vi "Run.vi"(8 "error in (no error)":errorcluster, 11 "socket PUB in":refnum<class "socket PUB.lvclass">) -> (0 "error out":errorcluster, 3 "socket PUB out":refnum<class "socket PUB.lvclass">)   [LabVIEW 2018, in "socket PUB.lvclass"]
uses:
  socket PUB.lvclass
  C:/Users/Denis/Desktop/S4ACS/S4ACS/communication-manager/Socket/Socket.lvclass
  State Machine/State Machine.lvclass
  RxTx/RxTx.lvclass
  Socket/Socket.lvclass
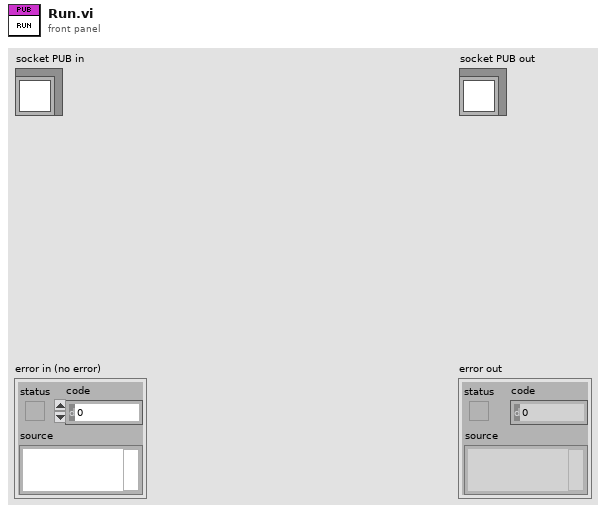
[diagram p1: front panel]
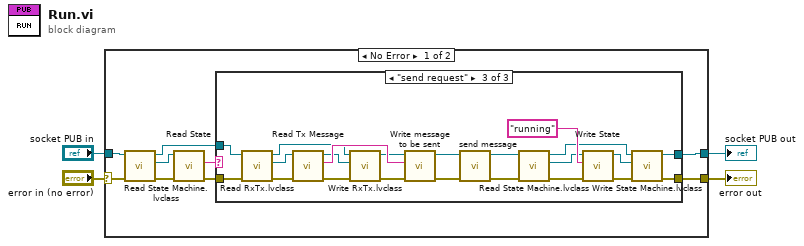
[diagram p0: block diagram]
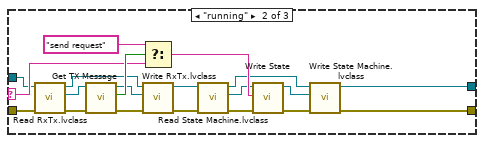
[diagram p3: hidden frame]
diagram:
  n1 = case shown="No Error" "error in (no error)" {
    selector: "error in (no error)" -> [w9 w58]
    tunnel: "socket PUB in" -> [w7 w59]
    tunnel: [w5 w59] -> w2
    tunnel: [w8 w58] -> w1
    frame No Error {
      n2 = call-dynamic "Read State Machine.lvclass.vi"("error in (no error)"=w9, "Socket in"=w7) -> ("error out"=w11:errorcluster, "State Machine.lvclass"=w13:refnum<class "State Machine.lvclass">, "Socket out"=w6:refnum<class "socket PUB.lvclass">)  [unwired: 7 in]
      n3 = call-dynamic "Read State.vi"("error in (no error)"=w11, "State Machine in"=w13) -> ("error out"=w10:errorcluster, "State"=w12:string)  [unwired: 7 in, 1 out]
      n4 = case shown="\"send request\"" w12 {
        selector: w12 -> [_ w34 _]
        tunnel: w6 -> [w15 w22 w54]
        tunnel: [w15 w16 w48] -> w5
        tunnel: [w14 w25 w47] -> w8
        tunnel: w10 -> [w14 w32 w53]
        frame Default {
        }
        frame "running" {
          n5 = call-dynamic "Read RxTx.lvclass.vi"("error in (no error)"=w32, "Socket in"=w22) -> ("error out"=w28:errorcluster, "RxTx.lvclass"=w30:refnum<class "RxTx.lvclass">, "Socket out"=w21:refnum<class "socket PUB.lvclass">)  [unwired: 7 in]
          n6 = call "Get TX Message.vi"("error in (no error)"=w28, "RxTx in"=w30) -> ("error out"=w27:errorcluster, "New msg"=w35:bool, "RxTx out"=w29:refnum<class "RxTx.lvclass">)  [unwired: 7 in]
          n7 = Select(t="send request", s=w35, f=w34) -> (s? t:f=w31:string)
          n8 = call-dynamic "Write RxTx.lvclass.vi"("error in (no error)"=w27, "RxTx.lvclass"=w29, "Socket in"=w21) -> ("error out"=w24:errorcluster, "Socket out"=w20:refnum<class "socket PUB.lvclass">)  [unwired: 7 in]
          n9 = call-dynamic "Read State Machine.lvclass.vi"("error in (no error)"=w24, "Socket in"=w20) -> ("error out"=w23:errorcluster, "State Machine.lvclass"=w18:refnum<class "State Machine.lvclass">, "Socket out"=w19:refnum<class "socket PUB.lvclass">)  [unwired: 7 in]
          n10 = call-dynamic "Write State.vi"("error in (no error)"=w23, "State"=w31, "State Machine in"=w18) -> ("error out"=w26:errorcluster, "State Machine out"=w17:refnum<class "State Machine.lvclass">)  [unwired: 7 in]
          n11 = call-dynamic "Write State Machine.lvclass.vi"("error in (no error)"=w26, "State Machine.lvclass"=w17, "Socket in"=w19) -> ("error out"=w25:errorcluster, "Socket out"=w16:refnum<class "socket PUB.lvclass">)  [unwired: 7 in]
        }
        frame "send request" {
          n12 = call-dynamic "Read RxTx.lvclass.vi"("error in (no error)"=w53, "Socket in"=w54) -> ("error out"=w38:errorcluster, "RxTx.lvclass"=w52:refnum<class "RxTx.lvclass">, "Socket out"=w43:refnum<class "socket PUB.lvclass">)  [unwired: 7 in]
          n13 = call "Read Tx Message.vi"("error in (no error)"=w38, "RxTx in"=w52) -> ("error out"=w40:errorcluster, "Tx Message"=w55:string, "RxTx out"=w39:refnum<class "RxTx.lvclass">)  [unwired: 7 in]
          n14 = call-dynamic "Write RxTx.lvclass.vi"("error in (no error)"=w40, "RxTx.lvclass"=w39, "Socket in"=w43) -> ("error out"=w41:errorcluster, "Socket out"=w42:refnum<class "socket PUB.lvclass">)  [unwired: 7 in]
          n15 = call-dynamic "Write message to be sent.vi"("error in (no error)"=w41, "message to be sent"=w55, "Socket in"=w42) -> ("error out"=w56:errorcluster, "Socket out"=w57:refnum<class "socket PUB.lvclass">)  [unwired: 7 in]
          n16 = call "send message.vi"("error in (no error)"=w56, "Socket in"=w57) -> ("error out"=w36:errorcluster, "Socket out"=w37:refnum<class "socket PUB.lvclass">)  [unwired: 8 in]
          n17 = call-dynamic "Read State Machine.lvclass.vi"("error in (no error)"=w36, "Socket in"=w37) -> ("error out"=w46:errorcluster, "State Machine.lvclass"=w45:refnum<class "State Machine.lvclass">, "Socket out"=w44:refnum<class "socket PUB.lvclass">)  [unwired: 7 in]
          n18 = call-dynamic "Write State.vi"("error in (no error)"=w46, "State"="running" ("new state"), "State Machine in"=w45) -> ("error out"=w49:errorcluster, "State Machine out"=w50:refnum<class "State Machine.lvclass">)  [unwired: 7 in]
          n19 = call-dynamic "Write State Machine.lvclass.vi"("error in (no error)"=w49, "State Machine.lvclass"=w50, "Socket in"=w44) -> ("error out"=w47:errorcluster, "Socket out"=w48:refnum<class "socket PUB.lvclass">)  [unwired: 7 in]
        }
      }
    }
    frame Error {
    }
  }
  "error out" <- w1
  "socket PUB out" <- w2
